vi "VIPM package Testing automation.vi"() -> ()   [LabVIEW 2016]
uses:
  <vilib>/addons/_JKI Toolkits/Caraya/classes/Test Result/Test Result.lvclass
panel:
  out "Passed ?":bool
  out "error out":errorcluster
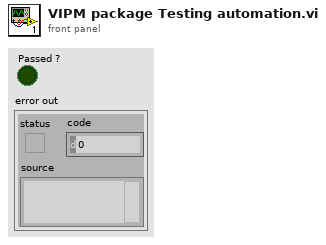
[diagram p1: front panel]
types:
  T1 = typedef "Caraya.lvlib/Test Result.lvclass/Node Results.ctl" = cluster{"Node":T2, "Assertions":T4[]}
  T2 = typedef "Caraya.lvlib/Test Result.lvclass/Test Node.ctl" = cluster{"Test Registration":T3, "Defined":bool, "Passed":bool}
  T3 = typedef "Caraya.lvlib/Test Result.lvclass/Test Registration Data.ctl" = cluster{"Name":string, "Call Chain":string[], "Time Stamp":timestamp, "Test ID":string, "Caller ID":string}
  T4 = typedef "Caraya.lvlib/Test Result.lvclass/Assert Event Data.ctl" = cluster{"Name":string, "Passed":bool, "Call Chain":string[], "Test Error":errorcluster, "Time Stamp":timestamp, "Unique Assert ID":string, "Test ID":string, "Execution time (s)":dbl, "Verbose Explanation":string}
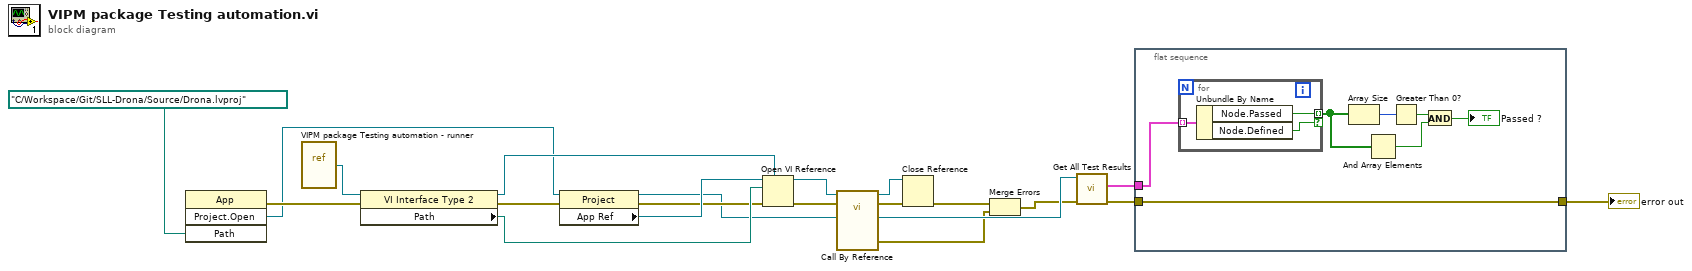
[diagram p0: block diagram]
diagram:
  n1 = invoke class="App" method="Project.Open"("Path"=path "C:/Workspace/Git/SLL-Drona/Source/Drona.lvproj") -> (error out=w13:errorcluster, "Project:Open"=w8:refnum<vi>)  [unwired: 3 in, 2 out]
  n2 = vi-ref "VIPM package Testing automation - runner.vi"() -> (w21:refnum<vi>)
  n3 = property class="VI Interface Type 2"(reference=w21, error in=w13) -> (reference out=w20:refnum<vi>, error out=w12:errorcluster, "Path"=w19:path)
  n4 = property class="Project"(reference=w8, error in=w12) -> (reference out=w10:refnum<vi>, error out=w11:errorcluster, "App Ref"=w14:refnum<vi>)
  n5 = Open VI Reference(type specifier VI Refnum (for type only)=w20, application reference (local)=w14, vi path=w19, error in (no error)=w11) -> (vi reference=w17:refnum<vi>, error out=w18:errorcluster)  [unwired: 2 in]
  n6 = call-by-ref "?"(reference=w17, error in=w18, "Project Refnum"=w10) -> (reference out=w15:refnum<vi>, error out=w16:errorcluster, 0:"error out"=w4:errorcluster, "Test Suite Results"=w7:refnum<class "Test Result.lvclass">)  [unwired: 9 in]
  n7 = Close Reference(reference=w15, error in (no error)=w16) -> (error out=w9:errorcluster)
  n8 = Merge Errors(w9, w4) -> (w5:errorcluster)
  n9 = call <vilib>:"Get All Test Results.vi"("error in (no error)"=w5, "Test Result in"=w7) -> ("error out"=w2:errorcluster, "Test Results"=w3:T1[])  [unwired: 7 in, 1 out]
  n10 = flat-sequence {
    tunnel: w3 -> [w28]
    tunnel: [w22] -> w1
    tunnel: w2 -> [w22]
    frame #0 {
      n11 = for {
        tunnel: w28 -> [w31] mode=indexing
        tunnel: [w30] -> w24 mode=indexing if=w29
        n12 = Unbundle By Name(w31) -> ("Node.Passed"=w30:bool, "Node.Defined"=w29:bool)
      }
      n13 = Array Size(array=w24) -> (size(s)=w27:i32)
      n14 = And Array Elements(Boolean array=w24) -> (logical AND=w25:bool)
      n15 = Greater Than 0?(x=w27) -> (x > 0?=w26:bool)
      n16 = And(x=w26, y=w25) -> (x .and. y?=→"Passed ?":bool)
    }
  }
  "error out" <- w1
